vi "subVI_init3CONEXactuators.vi"(3 "error in (no error)":errorcluster, 4 "Connected devices":string[](array[string])=["COM3", "COM4", "COM5"], 5 "Controller Addresses":i32[](array[numeric])=[1, 1, 1]) -> (0 "Error OUT":errorcluster, 2 "CONEX Cluster":T1)   [LabVIEW 2010]
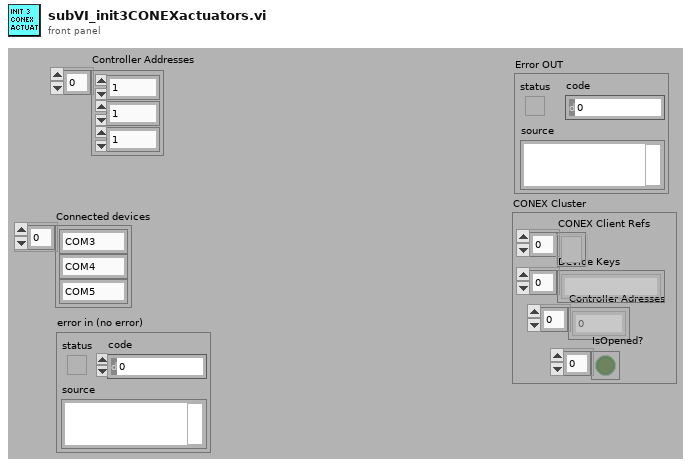
[diagram p1: front panel]
types:
  T1 = cluster{"CONEX Client Refs":refnum<k24>[], "Device Keys":string[], "Controller Adresses":i32[], "IsOpened?":bool[]}
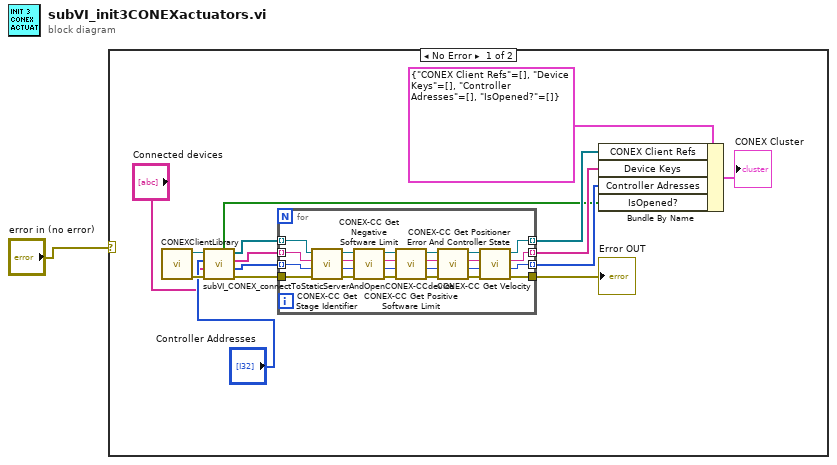
[diagram p0: block diagram]
diagram:
  n1 = case shown="No Error" "error in (no error)" {
    frame No Error {
      n2 = call <userlib>:"CONEXClientLibrary.vi"() -> ("CONEX Client LIB ref"=w16:refnum<k24>, "Error OUT"=w15:errorcluster)  [unwired: 4 in]
      n3 = call "subVI_CONEX_connectToStaticServerAndOpenCONEX-CCdevice.vi"("Error IN"=w15, "Connected devices"="Connected devices", "Controller Addresses"="Controller Addresses", "CONEX Client Lib Ref"=w16) -> ("error out"=w14:errorcluster, "Addresses out"=w11:i32[], "Device Keys Out"=w12:string[], "CONEX Client Refs out"=w13:refnum<k24>[], "IsOpened?"=w2:bool[])  [unwired: 2 in, 1 out]
      n4 = for {
        tunnel: w14 -> [w40]
        tunnel: w13 -> [w39] mode=indexing
        tunnel: w12 -> [w38] mode=indexing
        tunnel: w11 -> [w37] mode=indexing
        tunnel: [w20] -> w8 mode=indexing
        tunnel: [w19] -> w7 mode=indexing
        tunnel: [w18] -> w6 mode=indexing
        tunnel: [w17] -> w10
        n5 = call <userlib>:"CONEX-CC Get Stage Identifier.vi"("CONEX Client Ref IN"=w39, "deviceKey"=w38, "Address"=w37, "Error IN"=w40) -> ("CONEX Client Ref OUT"=w36:refnum<k24>, "deviceKey OUT"=w35:string, "Address OUT"=w34:i32, "Error OUT"=w33:errorcluster)  [unwired: 1 out]
        n6 = call <userlib>:"CONEX-CC Get Negative Software Limit.vi"("CONEX Client Ref IN"=w36, "deviceKey IN"=w35, "Address IN"=w34, "Error IN"=w33) -> ("CONEX Client Ref OUT"=w32:refnum<k24>, "deviceKey OUT"=w31:string, "Address OUT"=w30:i32, "Error OUT"=w29:errorcluster)  [unwired: 2 out]
        n7 = call <userlib>:"CONEX-CC Get Positive Software Limit.vi"("CONEX Client Ref IN"=w32, "deviceKey IN"=w31, "Address IN"=w30, "Error IN"=w29) -> ("CONEX Client Ref OUT"=w28:refnum<k24>, "deviceKey OUT"=w27:string, "Address OUT"=w26:i32, "Error OUT"=w25:errorcluster)  [unwired: 2 out]
        n8 = call <userlib>:"CONEX-CC Get Velocity.vi"("CONEX Client Ref IN"=w28, "deviceKey IN"=w27, "Address IN"=w26, "Error IN"=w25) -> ("CONEX Client Ref OUT"=w24:refnum<k24>, "deviceKey OUT"=w23:string, "Address OUT"=w22:i32, "Error OUT"=w21:errorcluster)  [unwired: 1 out]
        n9 = call <userlib>:"CONEX-CC Get Positioner Error And Controller State.vi"("CONEX Client Ref IN"=w24, "deviceKey"=w23, "Address IN"=w22, "Error IN"=w21) -> ("CONEX Client Ref OUT"=w20:refnum<k24>, "deviceKey OUT"=w19:string, "Address OUT"=w18:i32, "Error OUT"=w17:errorcluster)  [unwired: 2 out]
      }
      "Error OUT" <- w10
      n10 = Bundle By Name(cluster=T1 {"CONEX Client Refs"=[], "Device Keys"=[], "Controller Adresses"=[], "IsOpened?"=[]}, "CONEX Client Refs"=w8, "Device Keys"=w7, "Controller Adresses"=w6, "IsOpened?"=w2) -> (→"CONEX Cluster":T1)
    }
    frame Error {
    }
  }
